vi "Helper SubVI - Image Compression DBL.vi"(9 "bits":i32=1 min=1 max=64, 11 "2D DWT coef":T1(array[cluster])) -> (3 "compressed coef":T1(array[cluster]))   [LabVIEW 2023]
doc: "Uses entropy-based encoding techniques to reduce the bit rate of the wavelet coefficients and achieve image compression."
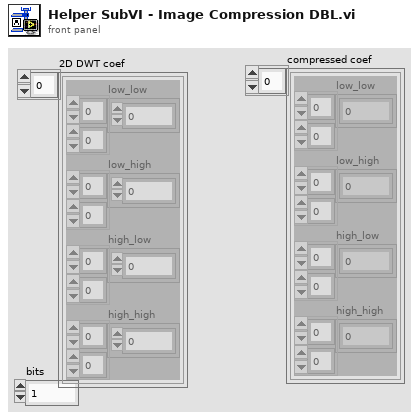
[diagram p1: front panel]
types:
  T1 = cluster{"low_low":dbl[][], "low_high":dbl[][], "high_low":dbl[][], "high_high":dbl[][]}[]
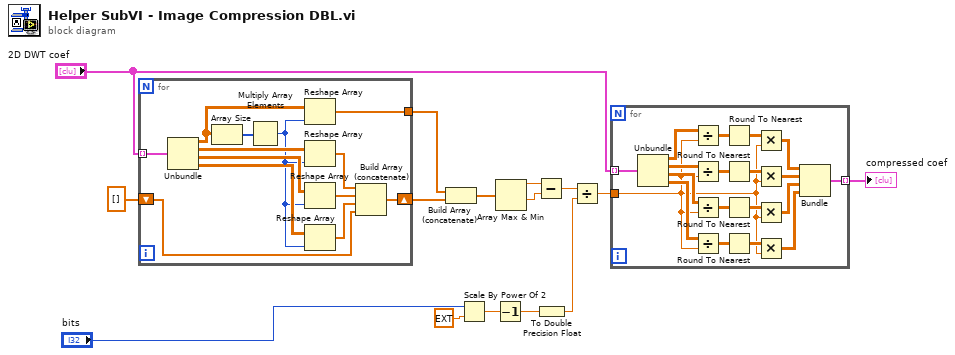
[diagram p0: block diagram]
diagram:
  n1 = for {
    tunnel: "2D DWT coef" -> [w28] mode=indexing
    tunnel: [w22] -> w14
    shift-right: [w21] -> w15
    shift-left: dbl[] [] -> [w19]
    n2 = Unbundle(w28) -> ("low_low"=w27:dbl[][], "low_high"=w25:dbl[][], "high_low"=w24:dbl[][], "high_high"=w23:dbl[][])
    n3 = Array Size(array=w27) -> (size(s)=w26:i32[])
    n4 = Multiply Array Elements(1:w26) -> (0:w16:i32)
    n5 = Reshape Array(w27, w16) -> (w22:dbl[])
    n6 = Reshape Array(w25, w16) -> (w18:dbl[])
    n7 = Reshape Array(w24, w16) -> (w17:dbl[])
    n8 = Reshape Array(w23, w16) -> (w20:dbl[])
    n9 = Build Array (concatenate)(w18, w17, w20, w19) -> (w21:dbl[])
  }
  n10 = Build Array (concatenate)(w14, w15) -> (w5:dbl[])
  n11 = Scale By Power Of 2(n="bits", x=ext 1.0) -> (x*2^n=w10:ext)
  n12 = Decrement(x=w10) -> (x-1=w11:ext)
  n13 = Array Max & Min(array=w5) -> (max value=w6:dbl, min value=w7:dbl)  [unwired: 2 out]
  n14 = Subtract(x=w6, y=w7) -> (x-y=w8:dbl)
  n15 = To Double Precision Float(number=w11) -> (double precision float=w12:dbl)
  n16 = Divide(x=w8, y=w12) -> (x/y=w3:dbl)
  n17 = for {
    tunnel: w3 -> [w34]
    tunnel: "2D DWT coef" -> [w47] mode=indexing
    tunnel: [w29] -> w1 mode=indexing
    n18 = Unbundle(w47) -> ("low_low"=w46:dbl[][], "low_high"=w37:dbl[][], "high_low"=w36:dbl[][], "high_high"=w35:dbl[][])
    n19 = Divide(x=w46, y=w34) -> (x/y=w45:dbl[][])
    n20 = Divide(x=w37, y=w34) -> (x/y=w42:dbl[][])
    n21 = Divide(x=w36, y=w34) -> (x/y=w41:dbl[][])
    n22 = Divide(x=w35, y=w34) -> (x/y=w38:dbl[][])
    n23 = Round To Nearest(number=w45) -> (nearest integer value=w44:dbl[][])
    n24 = Round To Nearest(number=w42) -> (nearest integer value=w43:dbl[][])
    n25 = Round To Nearest(number=w41) -> (nearest integer value=w40:dbl[][])
    n26 = Round To Nearest(number=w38) -> (nearest integer value=w39:dbl[][])
    n27 = Multiply(x=w44, y=w34) -> (x*y=w32:dbl[][])
    n28 = Multiply(x=w43, y=w34) -> (x*y=w33:dbl[][])
    n29 = Multiply(x=w40, y=w34) -> (x*y=w31:dbl[][])
    n30 = Multiply(x=w39, y=w34) -> (x*y=w30:dbl[][])
    n31 = Bundle(w32, w33, w31, w30) -> (w29:cluster{dbl[][], dbl[][], dbl[][], dbl[][]})  [unwired: 1 out]
  }
  "compressed coef" <- w1
